vi "Link Speed Test.vi"(8 "error in":errorcluster, 11 "XNET Interface":refnum<k21>="ENET1") -> (0 "error out":errorcluster, 3 "DUT Info":T1 {"Link Speed Configured" items=["100Mb/s"=100, "1000Mb/s"=1000]; "Sleep Capability Configured" items=["Disabled", "Enabled"]; "PHY State" items=["Slave", "Master"]; "Port Mode" items=["Direct", "Tap"]; "Jumbo Frames" items=["Disabled", "9018_bytes"]; "Interrupt Moderation" items=["Off", "Low", "Medium", "High"]})   [LabVIEW 2026]
uses:
  Device Info.ctl
  <vilib>/nisyscfg/Save Changes (Hardware).vi
  <vilib>/nisyscfg/Close (Resources).vi
  <vilib>/nisyscfg/Close (Filter).vi
  <vilib>/nisyscfg/Close (System).vi
  <vilib>/nisyscfg/nisyscfg.lvlib
  <resource>/objmgr/niflexrioatomicsae.rc
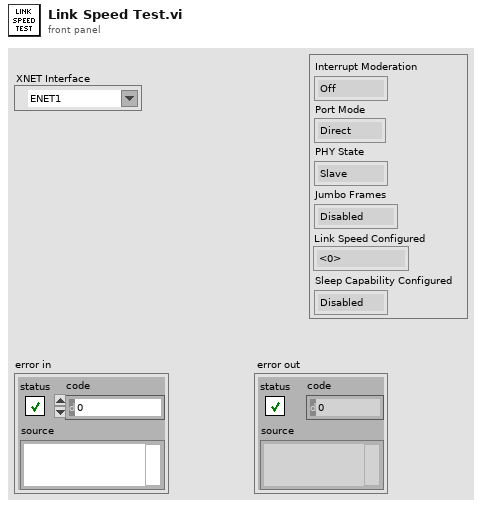
[diagram p1: front panel]
types:
  T1 = typedef "Device Info.ctl" = cluster{"Interrupt Moderation":u32, "Jumbo Frames":u32, "Port Mode":u32, "PHY State":u32, "Sleep Capability Configured":u32, "Link Speed Configured":u32}
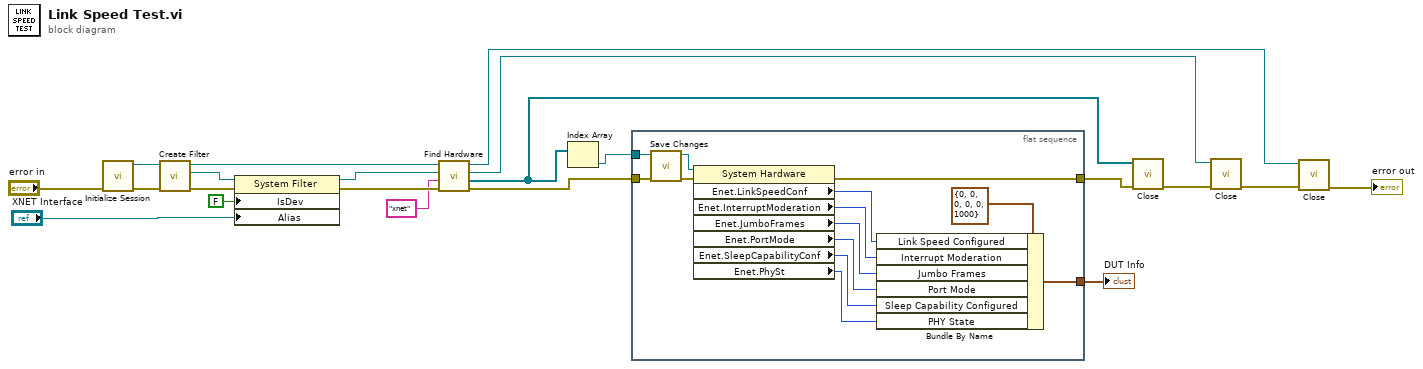
[diagram p0: block diagram]
diagram:
  n1 = call <vilib>:"Initialize Session.vi"("error in (no error)"="error in") -> ("error out"=w19:errorcluster, "Session out"=w18:refnum<k21>)  [unwired: 9 in]
  n2 = call <vilib>:"Create Filter.vi"("error in (no error)"=w19, "Session in"=w18) -> ("error out"=w21:errorcluster, "Filter out"=w20:refnum<k20>, "Session out"=w8:refnum<k21>)  [unwired: 7 in]
  n3 = property class="System Filter"(reference=w20, error in=w21, "IsDev"=FALSE ("Is Device"), "Alias"="XNET Interface") -> (reference out=w15:refnum<k20>, error out=w16:errorcluster)
  n4 = call <vilib>:"Find Hardware.vi"("error in (no error)"=w16, "Experts"="xnet", "Filter in"=w15, "Session in"=w8) -> ("error out"=w12:errorcluster, "Resources out"=w9:refnum<k20>[], "Filter out"=w4:refnum<k20>, "Session out"=w5:refnum<k21>)  [unwired: 4 in]
  n5 = Index Array(array=w9) -> (element=w13:refnum<k20>)  [unwired: 1 in]
  n6 = flat-sequence {
    tunnel: w13 -> [w34]
    tunnel: w12 -> [w33]
    tunnel: [w32] -> w7
    tunnel: [w23] -> w1
    frame #0 {
      n7 = call-poly <vilib>:"Save Changes.vi"("error in (no error)"=w33, "Resource in"=w34) -> ("error out"=w30:errorcluster, "Resource out"=w31:refnum<k20>)  [unwired: 6 in, 2 out]
      n8 = property class="System Hardware"(reference=w31, error in=w30) -> (error out=w32:errorcluster, "Enet.LinkSpeedConf"=w29:u32, "Enet.InterruptModeration"=w28:u32, "Enet.JumboFrames"=w27:u32, "Enet.PortMode"=w26:u32, "Enet.SleepCapabilityConf"=w25:u32, "Enet.PhySt"=w24:u32)  [unwired: 1 out]
      n9 = Bundle By Name(cluster=T1 {"Interrupt Moderation"=0, "Jumbo Frames"=0, "Port Mode"=0, "PHY State"=0, "Sleep Capability Configured"=0, "Link Speed Configured"=1000} ("DUT Info"), "Link Speed Configured"=w29, "Interrupt Moderation"=w28, "Jumbo Frames"=w27, "Port Mode"=w26, "Sleep Capability Configured"=w25, "PHY State"=w24) -> (w23:T1)
    }
  }
  n10 = call-poly <vilib>:"Close.vi"("error in (no error)"=w7, "Resources in"=w9) -> ("error out"=w10:errorcluster)  [unwired: 9 in]
  n11 = call-poly <vilib>:"Close.vi"("error in (no error)"=w10, "Filter in"=w4) -> ("error out"=w6:errorcluster)  [unwired: 9 in]
  n12 = call-poly <vilib>:"Close.vi"("error in (no error)"=w6, "Session in"=w5) -> ("error out"=→"error out":errorcluster)  [unwired: 9 in]
  "DUT Info" <- w1
